vi "NI Vision to Galvo Coordinates.vi"(8 "Pixels Per Edge Y":dbl=200.0, 9 "Pixels Per Edge X":dbl=200.0, 11 "ROI":T2) -> (3 "Scanning":T1 {"A(cluster)/B" max=1000 step=1; "B-scans (rings)" max=1000 step=1; "Fast Axis Amp" max=20 format="%#.2f"; "Slow Axis Amp" max=20 format="%#.2f"; "Slow Axis Offset" max=10 format="%#.2f"; "Fast Axis Offset" max=10 format="%#.2f"})   [LabVIEW 2014]
uses:
  Classes/Galvo/Scanning Cluster.ctl
  Classes/Galvo/Galvo.lvclass
panel:
  in  "Cluster Def":T1 {"A(cluster)/B" max=1000 step=1; "B-scans (rings)" max=1000 step=1; "Fast Axis Amp" max=20 format="%#.2f"; "Slow Axis Amp" max=20 format="%#.2f"; "Slow Axis Offset" max=10 format="%#.2f"; "Fast Axis Offset" max=10 format="%#.2f"}
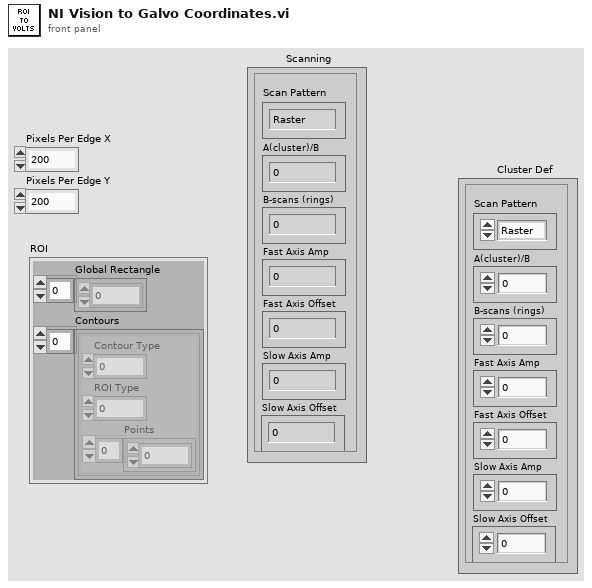
[diagram p1: front panel]
types:
  T1 = typedef "Galvo.lvclass/Scanning Cluster.ctl" = cluster{"Fast Axis Offset":sgl, "Slow Axis Offset":sgl, "Slow Axis Amp":sgl, "Fast Axis Amp":sgl, "B-scans (rings)":u32, "A(cluster)/B":u32, "Scan Pattern":enum16{"Raster"}}
  T2 = cluster{"Global Rectangle":i32[], "Contours":cluster{"Contour Type":u32, "ROI Type":u32, "Points":i32[]}[]}
  T3 = cluster{"Contour Type":u32, "ROI Type":u32, "Points":i32[]}[]
  T4 = cluster{"Contour Type":u32, "ROI Type":u32, "Points":i32[]}
  T5 = typedef "IMAQ Point" = cluster{"X":sgl, "Y":sgl}
  T6 = typedef "IMAQ Line" = cluster{"Start X":i32, "Start Y":i32, "End X":i32, "End Y":i32}
  T7 = typedef "IMAQ Rectangle" = cluster{"Left":i32, "Top":i32, "Right":i32, "Bottom":i32, "Rotation":dbl}
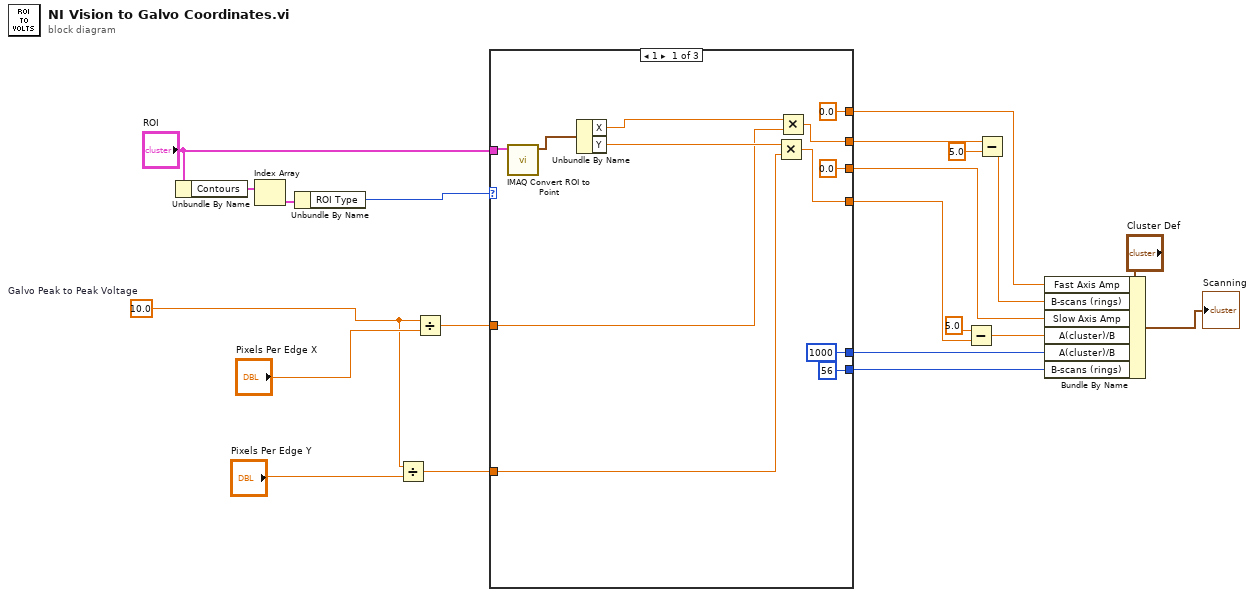
[diagram p0: block diagram]
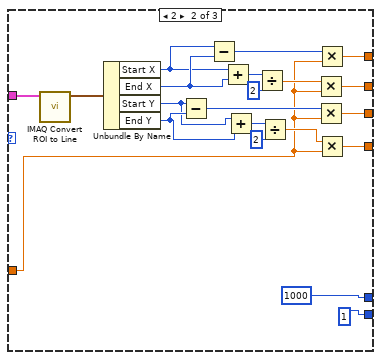
[diagram p2: hidden frame]
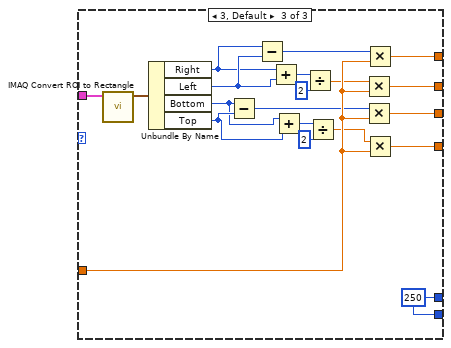
[diagram p3: hidden frame]
diagram:
  w2 = 10.0  # Galvo Peak to Peak Voltage
  n1 = Unbundle By Name("ROI") -> ("Contours"=w8:T3)
  n2 = Index Array(array=w8) -> (element=w7:T4)  [unwired: 1 in]
  n3 = Unbundle By Name(w7) -> ("ROI Type"=w6:u32)
  n4 = Divide(x=w2, y="Pixels Per Edge Y") -> (x/y=w1:dbl)
  n5 = Divide(x=w2, y="Pixels Per Edge X") -> (x/y=w13:dbl)
  n6 = case shown="1" w6 {
    tunnel: [w27 w39 w74] -> w21
    tunnel: [w28 w37 w73] -> w16
    tunnel: [0.0 w38 w72] -> w15
    tunnel: [0.0 w36 w71] -> w14
    tunnel: w13 -> [w29 w40 w70]
    tunnel: "ROI" -> [w33 w54 w56]
    tunnel: [1000 ("y") 1000 ("y") w55] -> w5
    tunnel: [56 ("y") 1 ("y") w55] -> w4
    tunnel: w1 -> [w22 _ _]
    frame 1 {
      n7 = call "IMAQ Convert ROI to Point"("ROI Descriptor"=w33) -> ("Point"=w32:T5)  [unwired: 8 in, 1 out]
      n8 = Unbundle By Name(w32) -> ("X"=w31:sgl, "Y"=w30:sgl)
      n9 = Multiply(x=w30, y=w22) -> (x*y=w27:dbl)
      n10 = Multiply(x=w31, y=w29) -> (x*y=w28:dbl)
    }
    frame 2 {
      n11 = call "IMAQ Convert ROI to Line"("ROI Descriptor"=w54) -> ("Line"=w41:T6)  [unwired: 8 in, 1 out]
      n12 = Unbundle By Name(w41) -> ("Start X"=w42:i32, "End X"=w43:i32, "Start Y"=w48:i32, "End Y"=w49:i32)
      n13 = Subtract(x=w48, y=w49) -> (x-y=w52:i32)
      n14 = Subtract(x=w42, y=w43) -> (x-y=w50:i32)
      n15 = Add(x=w42, y=w43) -> (x+y=w44:i32)
      n16 = Add(x=w48, y=w49) -> (x+y=w47:i32)
      n17 = Divide(x=w44, y=2) -> (x/y=w53:dbl)
      n18 = Divide(x=w47, y=2) -> (x/y=w51:dbl)
      n19 = Multiply(x=w53, y=w40) -> (x*y=w37:dbl)
      n20 = Multiply(x=w52, y=w40) -> (x*y=w38:dbl)
      n21 = Multiply(x=w50, y=w40) -> (x*y=w36:dbl)
      n22 = Multiply(x=w51, y=w40) -> (x*y=w39:dbl)
    }
    frame 3, Default {
      w55 = 250 ("y")
      n23 = call "IMAQ Convert ROI to Rectangle"("ROI Descriptor"=w56) -> ("Rectangle"=w57:T7)  [unwired: 8 in, 1 out]
      n24 = Unbundle By Name(w57) -> ("Right"=w58:i32, "Left"=w59:i32, "Bottom"=w64:i32, "Top"=w65:i32)
      n25 = Subtract(x=w64, y=w65) -> (x-y=w68:i32)
      n26 = Subtract(x=w58, y=w59) -> (x-y=w66:i32)
      n27 = Add(x=w58, y=w59) -> (x+y=w60:i32)
      n28 = Add(x=w64, y=w65) -> (x+y=w63:i32)
      n29 = Divide(x=w60, y=2) -> (x/y=w69:dbl)
      n30 = Divide(x=w63, y=2) -> (x/y=w67:dbl)
      n31 = Multiply(x=w69, y=w70) -> (x*y=w73:dbl)
      n32 = Multiply(x=w68, y=w70) -> (x*y=w72:dbl)
      n33 = Multiply(x=w66, y=w70) -> (x*y=w71:dbl)
      n34 = Multiply(x=w67, y=w70) -> (x*y=w74:dbl)
    }
  }
  n35 = Subtract(x=5.0 ("y"), y=w21) -> (x-y=w20:dbl)
  n36 = Subtract(x=w16, y=5.0) -> (x-y=w18:dbl)
  n37 = Bundle By Name(cluster="Cluster Def", "Fast Axis Amp"=w14, "B-scans (rings)"=w18, "Slow Axis Amp"=w15, "A(cluster)/B"=w20, "A(cluster)/B"=w5, "B-scans (rings)"=w4) -> (→"Scanning":T1)
